vi "getGlyphFile.vi"(8 "error in (no error)":errorcluster, 11 "DMA_Read in":refnum<class "DMA_Read.lvclass">) -> (0 "error out":errorcluster, 2 "Glyph File":string, 3 "DMA_Read out":refnum<class "DMA_Read.lvclass">)   [LabVIEW 2013, in "DMA_Read.lvclass"]
doc: "Dynamic Dispatch VI. Returns the name of the glyph file to be used as a glyph in the tree control. A empty string means no glyph."
uses:
  DMA_Read.lvclass
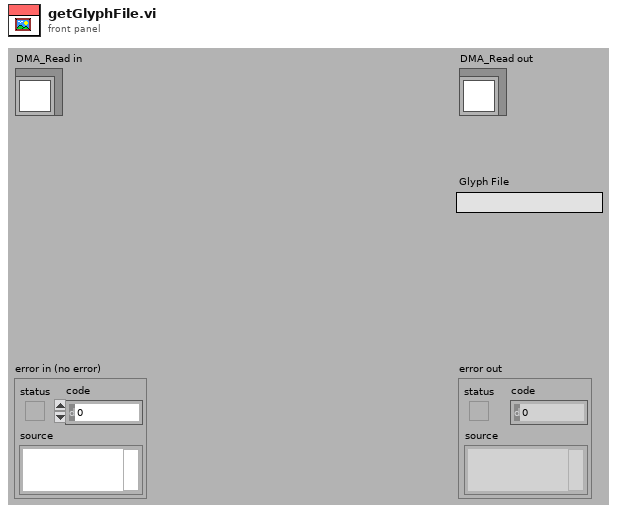
[diagram p1: front panel]
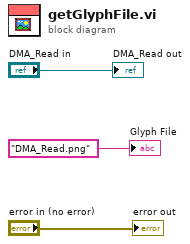
[diagram p0: block diagram]
diagram:
  "error out" <- "error in (no error)"
  "DMA_Read out" <- "DMA_Read in"
  "Glyph File" <- "DMA_Read.png" ("Glyph File")
